vi "Get_odour_data.vi"(3 "error in (no error)":errorcluster, 5 "Distance metric":string(combo)) -> (0 "error out":errorcluster, 2 "Odour component data":T1)   [LabVIEW 2016]
uses:
  <vilib>/Utility/file.llb/Read Delimited Spreadsheet (string).vi
  <vilib>/Utility/file.llb/Read Delimited Spreadsheet (DBL).vi
panel:
  out "2D map":dbl[][](array[numeric])
  out "volatility":dbl[](array[numeric])
  out "names":string[](array[string])
  out "CID":i32[](array[numeric])
  out "descriptors":string[][](array[string])
  out "distance matrix":dbl[][](array[numeric])
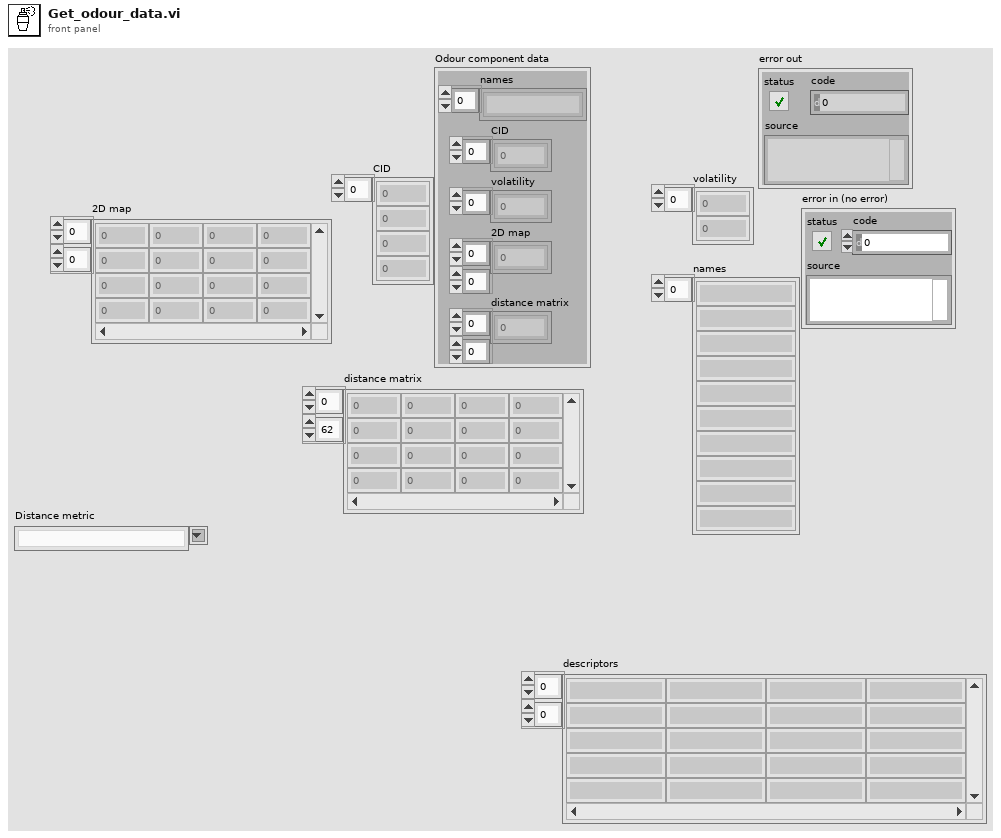
[diagram p1: front panel]
types:
  T1 = cluster{"names":string[], "CID":i32[], "volatility":dbl[], "2D map":dbl[][], "distance matrix":dbl[][]}
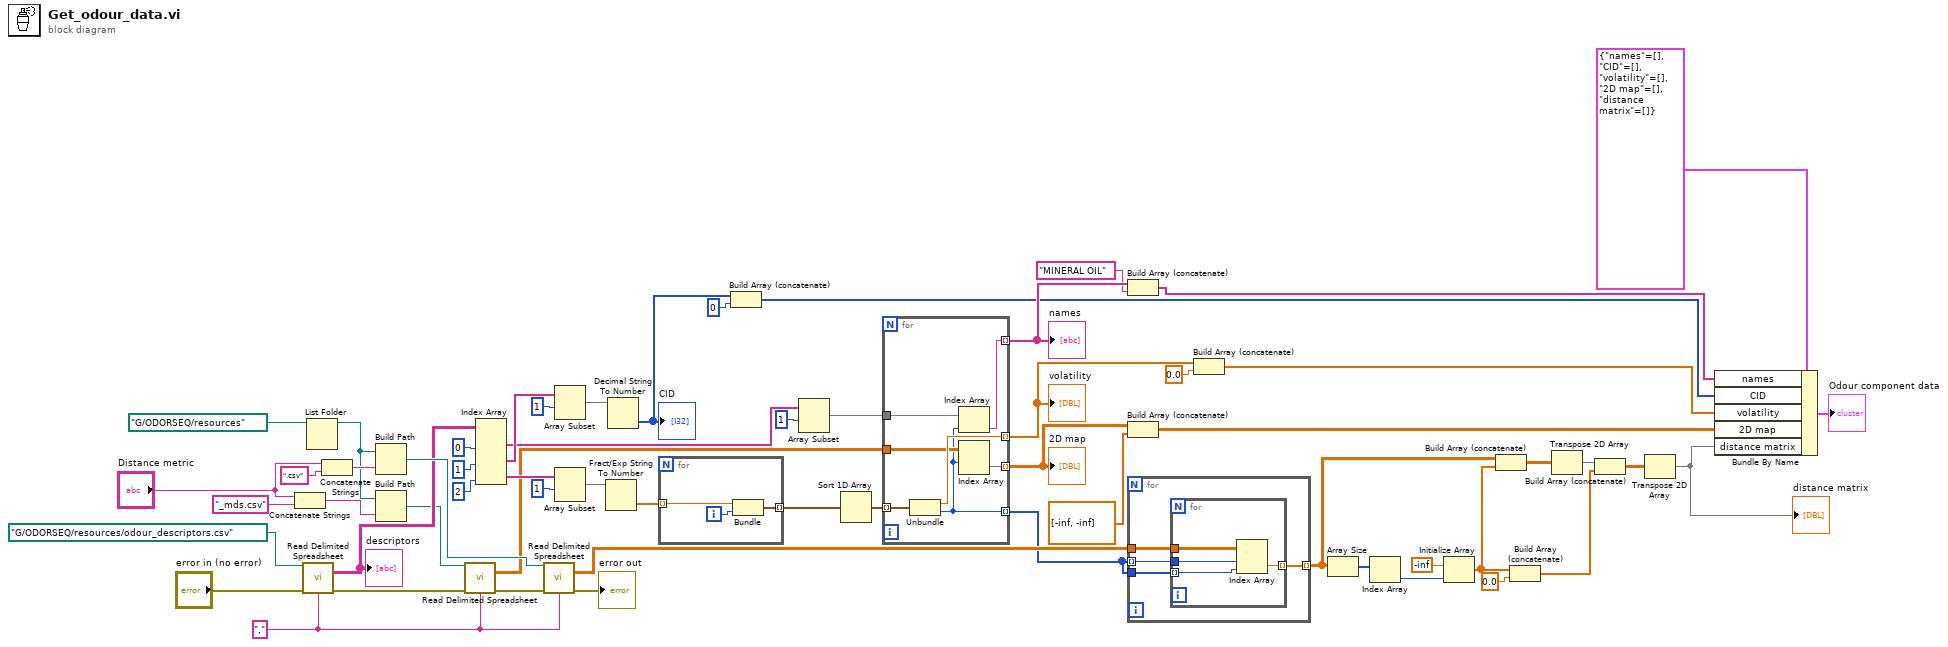
[diagram p0: block diagram]
diagram:
  w37 = "," ("delimiter (\\t)")
  n1 = Concatenate Strings("Distance metric", "_mds.csv" ("string")) -> (w41:string)
  n2 = call-poly <vilib>:"Read Delimited Spreadsheet.vi"("file path (dialog if empty)"=path "G:/ODORSEQ/resources/odour_descriptors.csv" ("Path"), "error in (no error)"="error in (no error)", "delimiter (\\t)"=w37) -> ("all rows"=w54:string[][], "error out"=w35:errorcluster)  [unwired: 7 in, 4 out]
  "descriptors" <- w54
  n3 = List Folder(path=path "G:/ODORSEQ/resources" ("Path")) -> (path out=w40:path)  [unwired: 3 in, 3 out]
  n4 = Concatenate Strings("Distance metric", ".csv" ("string")) -> (w58:string)
  n5 = Build Path(base path=w40, name or relative path=w58) -> (appended path=w56:path)
  n6 = Build Path(base path=w40, name or relative path=w41) -> (appended path=w38:path)
  n7 = call-poly <vilib>:"Read Delimited Spreadsheet.vi"("file path (dialog if empty)"=w38, "error in (no error)"=w35, "delimiter (\\t)"=w37) -> ("all rows"=w27:dbl[][], "error out"=w34:errorcluster)  [unwired: 7 in, 4 out]
  n8 = Index Array(array=w54, index (col) #1=0 ("disabled index (col)"), index (col) #2=1 ("disabled index (col)"), index (col) #3=2 ("index (col)")) -> (element #1=w48:string[], element #2=w50:string[], element #3=w44:string[])  [unwired: 3 in]
  n9 = call-poly <vilib>:"Read Delimited Spreadsheet.vi"("file path (dialog if empty)"=w56, "error in (no error)"=w34, "delimiter (\\t)"=w37) -> ("all rows"=w26:dbl[][], "error out"=→"error out":errorcluster)  [unwired: 7 in, 4 out]
  n10 = Array Subset(array=w50, index=1) -> (w52:string[])  [unwired: 1 in]
  n11 = Array Subset(array=w44, index=1) -> (w43:string[])  [unwired: 1 in]
  n12 = Fract/Exp String To Number(string=w43) -> (number=w31:dbl[])  [unwired: 3 in, 1 out]
  n13 = Decimal String To Number(string=w52) -> (number=w20:i32[])  [unwired: 2 in, 1 out]
  "CID" <- w20
  n14 = for {
    tunnel: w31 -> [w61] mode=indexing
    tunnel: [w62] -> w30 mode=indexing
    i -> [w60]
    n15 = Bundle("String"=w61, w60) -> (w62:cluster{"String":dbl, i32})  [unwired: 1 in]
  }
  n16 = Build Array (concatenate)(w20, 0) -> (w19:i32[])
  n17 = Array Subset(array=w48, index=1) -> (w28:string[])  [unwired: 1 in]
  n18 = Sort 1D Array(array=w30) -> (sorted array=w29:cluster{"String":dbl, i32}[])
  n19 = for {
    tunnel: w29 -> [w69] mode=indexing
    tunnel: [w68] -> w17 mode=indexing
    tunnel: w28 -> [w67]
    tunnel: [w66] -> w24 mode=indexing
    tunnel: w27 -> [w65]
    tunnel: [w64] -> w14 mode=indexing
    tunnel: [w63] -> w25 mode=indexing
    n20 = Unbundle(w69) -> ("String"=w68:dbl, w63:i32)
    n21 = Index Array(array=w67, index=w63) -> (element=w66:string)
    n22 = Index Array(array=w65, index (row)=w63) -> (element=w64:dbl[])  [unwired: 1 in]
  }
  "names" <- w24
  "volatility" <- w17
  "2D map" <- w14
  n23 = Build Array (concatenate)(w24, "MINERAL OIL") -> (w22:string[])
  n24 = Build Array (concatenate)(w14, dbl[] [-inf, -inf]) -> (w13:dbl[][])
  n25 = for {
    tunnel: w25 -> [w72] mode=indexing
    tunnel: w26 -> [w71]
    tunnel: w25 -> [w73]
    tunnel: [w70] -> w10 mode=indexing
    n26 = for {
      tunnel: w73 -> [w75] mode=indexing
      tunnel: w72 -> [w76]
      tunnel: w71 -> [w77]
      tunnel: [w74] -> w70 mode=indexing
      n27 = Index Array(array=w77, index (row)=w76, index (col)=w75) -> (element=w74:dbl)
    }
  }
  n28 = Build Array (concatenate)(w17, 0.0) -> (w16:dbl[])
  n29 = Array Size(array=w10) -> (size(s)=w11:i32[])
  n30 = Index Array(array=w11) -> (element=w8:i32)  [unwired: 1 in]
  n31 = Initialize Array(-inf, w8) -> (w5:dbl[])
  n32 = Build Array (concatenate)(w10, w5) -> (w7:dbl[][])
  n33 = Build Array (concatenate)(w5, 0.0 ("element")) -> (w3:dbl[])
  n34 = Transpose 2D Array(2D array=w7) -> (transposed array=w4:dbl[][])
  n35 = Build Array (concatenate)(w4, w3) -> (w2:dbl[][])
  n36 = Transpose 2D Array(2D array=w2) -> (transposed array=w1:dbl[][])
  "distance matrix" <- w1
  n37 = Bundle By Name(cluster=T1 {"names"=[], "CID"=[], "volatility"=[], "2D map"=[], "distance matrix"=[]}, "names"=w22, "CID"=w19, "volatility"=w16, "2D map"=w13, "distance matrix"=w1) -> (→"Odour component data":T1)
